vi "EcPlano.vi"(10 "MedicionesPuntos":dbl[][](array[numeric])) -> (2 "coeficientes":dbl[](array[numeric]))   [LabVIEW 2018]
uses:
  <vilib>/Analysis/NI_AALPro.lvlib
panel:
  out "Arreglo":dbl[](array[numeric])
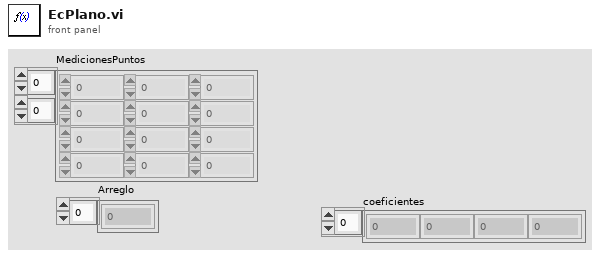
[diagram p1: front panel]
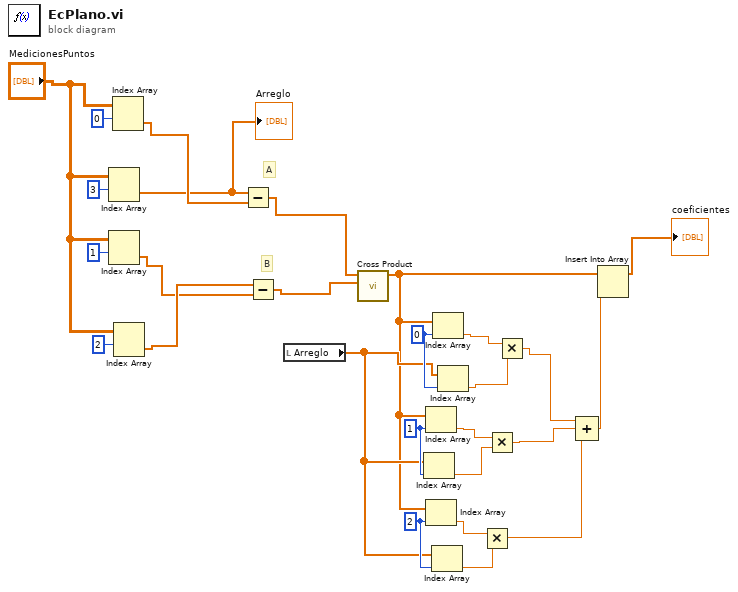
[diagram p0: block diagram]
diagram:
  w16 = 2 ("index (row)")
  w17 = 1 ("index (row)")
  w22 = 0 ("index (row)")
  # "B"
  # "A"
  n1 = Index Array(array="MedicionesPuntos", index (row)=3) -> (element=w1:dbl[])  [unwired: 1 in]
  "Arreglo" <- w1
  n2 = Index Array(array="MedicionesPuntos", index (row)=1) -> (element=w2:dbl[])  [unwired: 1 in]
  n3 = Index Array(array="MedicionesPuntos", index (row)=0) -> (element=w5:dbl[])  [unwired: 1 in]
  n4 = Index Array(array="MedicionesPuntos", index (row)=2) -> (element=w6:dbl[])  [unwired: 1 in]
  n5 = Subtract(x=w1, y=w5) -> (x-y=w24:dbl[])
  n6 = Subtract(x=w6, y=w2) -> (x-y=w23:dbl[])
  n7 = local read "Arreglo"() -> (w15:dbl[])
  n8 = call <vilib>:"Cross Product.vi"("B Vector"=w23, "A Vector"=w24) -> ("Cross Product"=w9:dbl[])  [unwired: 8 in, 1 out]
  n9 = Index Array(array=w15, index=w17) -> (element=w18:dbl)
  n10 = Index Array(array=w9, index=w17) -> (element=w19:dbl)
  n11 = Index Array(array=w9, index=w16) -> (element=w14:dbl)
  n12 = Index Array(array=w15, index=w16) -> (element=w13:dbl)
  n13 = Index Array(array=w9, index=w22) -> (element=w21:dbl)
  n14 = Index Array(array=w15, index=w22) -> (element=w20:dbl)
  n15 = Multiply(x=w14, y=w13) -> (x*y=w10:dbl)
  n16 = Multiply(x=w19, y=w18) -> (x*y=w11:dbl)
  n17 = Multiply(x=w21, y=w20) -> (x*y=w12:dbl)
  n18 = Compound Arithmetic op=ADD(w12, w11, w10) -> (w8:dbl)
  n19 = Insert Into Array(array=w9, new element=w8) -> (→"coeficientes":dbl[])  [unwired: 1 in]
